vi "HEWH Summary Sheet.vi"(6 "FHD Input":T2={"Calculated Values"={"Draw Cluster - Actual (Gal)"=[], "Mass of water All (lbm)"=[], "Density of hot water All (lbm/gal)"=[], "CpHW (BTU/(lbm °F))"=[], "rho 2 (lb/gal)"=0.0, "rho standby (lb/gal)"=0.0, "rho 24 (lb/gal)"=0.0, "Cp1 (BTU/(lb*F))"=0.0, "Cp2 (BTU/(lb*F))"=0.0, "Cp standby (BTU/(lb*F))"=0.0, "Cp 24 (BTU/(lb*F))"=0.0, "nu_r"=0.0, "Qstby (BTU)"=0.0, "Qhr (BTU/hr)"=0.0, "UA (BTU/(hr*F))"=0.0, "Q (BTU)"=0.0, "Qd (BTU)"=0.0, "Qda (BTU)"=0.0, "QHW67 (BTU)"=0.0, "UEF"=0.0, "Tdel1-Mean Outlet 1st Cluster(°F)"=0.0, "Tin1 - Mean Inlet 1st Cluster (°F)"=0.0, "Cp theoretical (BTU/(lbm °F))"=0.0, "M cluster mass removed (lb)"=0.0, "V1- Vol (Gal)"=0.0, "Test Data -Start to End (Full Index)"=[], "rho_nu (lb/gal)"=0.0, "Density of cold water All (lbm/gal)"=[], "CpUEF (BTU/(lb*F))"=0.0, "QHW (BTU)"=0.0, "QHWD (BTU)"=0.0, "Qdm (BTU)"=0.0, "FHD-After 1 Hour (String)"=[], "Vn"=0.0, "T*avg_del(n)"=0.0, "Max Location"=0, "T*min(n-1)"=0.0, "T*avg_del(n-1)"=0.0, "Temp Greater than T*min(n-1)"=FALSE, "Adjustment Factor"=0.0, "Draw Bonus Volume (gal)"=0.0, "Flow Type - End Condition"=enum."ForcedDrawAfterHour"}, "Sampled Data"={"Cold Water Draw Amounts-(Gal)"=[], "T del_all - Outlet Temps (°F)"=[], "T in_all - Inlet Temps (°F)"=[], "Qsu0 (BTU)"=14385.3, "Qsuf (BTU)"=15959.6, "Tau stby_1 (hr)"=8.4, "T suf(°F)"=125.0, "T su0(°F)"=126.1, "T tstby(°F)"=124.2, "T astby(°F)"=68.8, "T 24(°F)"=123.2, "Qr (BTU)"=7657.9, "T0 (°F)"=124.7, "Tmax1 (°F)"=124.8, "Qe (BTU)"=32770.2, "Qf (BTU)"=0.0, "Tastby2 (°F)"=68.9, "RTD Out Full Data\nSet (Each Draw)"=[], "RTD IN Full Data\nSet (Each Draw)"=[], "Tau stby2 (hr)"=23.406, "Hot Water Draw Amounts-(Gal)"=[], "Cold Flow Rate (GPM)"=[], "Hot Flow Rate (GPM)"=[], "Softw Elapsed Time\n Full Data Set (Each Draw)"=[], "Cold Gal Total Full\nData Set (Each Draw)"=[], "Total Hot Draw Amount (Gal) "=0.0, "Total Cold Draw Amount (Gal)"=0.0, "Qe (Wh)"=0.0, "Hot Gal Total Full\nData Set (Each Draw)"=[]}, "Static Data"={"T-Wh Setpoint (°F)"=125.0, "T-Inlet Setpoint (°F)"=58.0, "T-Ambinet Nominal (°F)"=67.5, "V - Volume of Wh (True)"=46.0}, "Data Indexes"={"Test Start-Full Index (Found)"=0, "Header Length"=0, "Draw Index (Found)"=[], "Nr"=0, "Start Watt Hours"=0.0, "Tsu0 Index (Found)"=0, "Tsf Index (Found)"=0, "Start Energy (BTU-Gas)"=0.0, "Draws in Cluster"=0, "T0 Index-Full Index (Found)"=0, "Non-Draw Index (Found)"=[], "Tmax1 Index (Found)"=0, "Test End-Full Index (Found)"=0, "Heating Index (Found)"=[], "Heating Timestamp"=[], "Non-Draw Timestamp"=[], "Draw Index Timestamp"=[], "Tmax1 Timestamp"=0.0, "Tsu0 Timestamp"=0.0, "Tsf Timestamp"=0.0, "T0 Timestamp"=0.0, "Test End Timestamp"=0.0, "Test Start Timestamp"=0.0, "15 sec after Draw Timestamp"=[], "15 sec after Draw Index"=[], "Tmax1 Occurred During a Draw"=FALSE, "FHD Total Time (Sec)"=0.0, "Draw Pattern"=enum."Very Small Usage", "Standby Valid"=FALSE}, "Raw Data"={"Elapsed Time Index (DBL)"=0, "Software Elapsed Time Index (DBL)"=0, "TC Tree Avg Index (DBL)"=0, "Watt Hours -Wh Index (DBL)"=0, "Energy BTU Index (DBL)"=0, "Totalized Flow Index (DBL)"=0, "Flow Rate Index (DBL)"=0, "Program Status Index (Str)"=0, "RTDin Index (DBL)"=0, "RTDout Index (DBL)"=0, "RTDamb Index (DBL)"=0, "Test Data-Start to End DBL"=[], "Data Type"=enum."GEA Inlet Side Meter", "Heat Source Index (DBL)"=0, "Hot Water Rate GPM (DBL)"=0, "Hot Water Total - GAL (DBL)"=0, "FHD-After 1 hour"=[], "Humidity -% RH (DBL)"=0, "Voltage - V (DBL)"=0, "Draw Count (DBL)"=0, "Elapsed Time Index (Str)"=0, "Software Elapsed Time Index (Str)"=0, "Frequency-Hz (Str)"=0, "RTDin Index (Str)"=0, "RTDout Index (Str)"=0, "RTDamb Index (Str)"=0, "UE (Str)"=0, "LE (Str)"=0, "Compressor (Str)"=0, "Flow Rate Index (Str)"=0, "Hot Water Total - GAL (Str)"=0}, "Tolerance Check (T)=Pass"={"Flow Rate"=FALSE, "Totalized Flow"=FALSE, "Ambient Temp (Full Range)"=FALSE, "Ambient Humidity (Full Range)"=FALSE, "Inlet Temp"=FALSE, "Outlet Temp"=FALSE, "Valid Test"=FALSE, "Individual Totalized Flow"=FALSE, "Data Sheet Check"="", "Inlet Temperature"=[], "Tinlet Max"=[], "Tinlet Min"=[], "Flow Rate Max (Tol)"=[], "Flow Rate Min (Tol)"=[], "Amb Temp Max"=0.0, "Amb Temp Min"=0.0, "Toutlet Max - Draw 1"=0.0, "Humidity Upper Tolerance (%)"=0.0, "Total Volume Tolerance (Gal)"=0.0, "Humidity Lower Tolerance (%)"=0.0, "Flow Rate Max\nPer Draw"=[], "Flow Rate Min\nPer Draw"=[], "Ambient Humidity (Runtime)"=FALSE, "Humidity Avg (Runtime)"=0.0, "Ambient Temp (On-Time AVG)"=FALSE, "Ambient Temp (Off-Time AVG)"=FALSE, "Amb Temp OFF Avg"=0.0, "Amb Temp ON Avg"=0.0, "Voltage (Heating)"=FALSE, "Voltage (Min)"=0.0, "Voltage (Max)"=0.0, "Toutlet Max"=[], "Toutlet Min"=[]}, "Test Information"={"TR Number"="", "Lab ID"="", "Notes/Config"="", "Model Number"="", "Serial Number"="", "Lab Technician"="", "Engineer"="", "Type of Fuel"="", "Samp Received Date"="", "Samp Test Date"="", "Report Date"="", "Rate Input (kW or BTU/hr)"="", "Measured Input (kW or BTU/hr)"="", "Filename"="", "Calibration Information"=[], "Calculator Version"="", "Minimum UEF Per CFR"=0.0, "UEF Report Information"=[], "FHR Report Information"=[], "FHR Front Panel Display"=[], "UEF Front Panel Display"=[], "Draw Outlet Temp Viewer"=[]}} {"Data Indexes"."15 sec after Draw Index" format="%#.2f"; "Data Indexes"."15 sec after Draw Timestamp" format="%#.2f"; "Data Indexes"."Test Start Timestamp" format="%.2f"; "Data Indexes"."Test End Timestamp" format="%.2f"; "Data Indexes"."T0 Timestamp" format="%.2f"; "Data Indexes"."Tsf Timestamp" format="%.2f"; "Data Indexes"."Tsu0 Timestamp" format="%.2f"; "Data Indexes"."Tmax1 Timestamp" format="%.2f"; "Data Indexes"."Draw Index Timestamp" format="%#.2f"; "Data Indexes"."Non-Draw Timestamp" format="%#.2f"; "Data Indexes"."Heating Timestamp" format="%#.2f"; "Data Indexes"."Start Energy (BTU-Gas)" format="%.6f"; "Data Indexes"."Start Watt Hours" format="%.6f"; "Static Data"."V - Volume of Wh (True)" format="%.5f"; "Static Data"."T-Ambinet Nominal (°F)" format="%.5f"; "Static Data"."T-Inlet Setpoint (°F)" format="%.5f"; "Static Data"."T-Wh Setpoint (°F)" format="%.5f"; "Sampled Data"."Qe (Wh)" format="%.5f"; "Sampled Data"."Tau stby2 (hr)" format="%.5f"; "Sampled Data"."Tastby2 (°F)" format="%.5f"; "Sampled Data"."Qf (BTU)" format="%.5f"; "Sampled Data"."Qe (BTU)" format="%.5f"; "Sampled Data"."Tmax1 (°F)" format="%.5f"; "Sampled Data"."T0 (°F)" format="%.5f"; "Sampled Data"."Qr (BTU)" format="%.5f"; "Sampled Data"."T 24(°F)" format="%.5f"; "Sampled Data"."T astby(°F)" format="%.5f"; "Sampled Data"."T tstby(°F)" format="%.5f"; "Sampled Data"."T su0(°F)" format="%.5f"; "Sampled Data"."T suf(°F)" format="%.5f"; "Sampled Data"."Tau stby_1 (hr)" format="%.5f"; "Sampled Data"."Qsuf (BTU)" format="%.5f"; "Sampled Data"."Qsu0 (BTU)" format="%.5f"; "Calculated Values"."Draw Bonus Volume (gal)" format="%.6f"; "Calculated Values"."Adjustment Factor" format="%.6f"; "Calculated Values"."T*avg_del(n-1)" format="%.6f"; "Calculated Values"."T*min(n-1)" format="%.6f"; "Calculated Values"."T*avg_del(n)" format="%.6f"; "Calculated Values"."Vn" format="%.6f"; "Calculated Values"."Qdm (BTU)" format="%.6f"; "Calculated Values"."QHWD (BTU)" format="%.6f"; "Calculated Values"."QHW (BTU)" format="%.6f"; "Calculated Values"."UEF" format="%.6f"; "Calculated Values"."QHW67 (BTU)" format="%.6f"; "Calculated Values"."Qda (BTU)" format="%.6f"; "Calculated Values"."Qd (BTU)" format="%.6f"; "Calculated Values"."Q (BTU)" format="%.6f"; "Calculated Values"."UA (BTU/(hr*F))" format="%.6f"; "Calculated Values"."Qhr (BTU/hr)" format="%.6f"; "Calculated Values"."Qstby (BTU)" format="%.6f"; "Calculated Values"."nu_r" format="%.6f"; "Calculated Values"."CpUEF (BTU/(lb*F))" format="%.6f"; "Calculated Values"."rho_nu (lb/gal)" format="%.6f"; "Calculated Values"."V1- Vol (Gal)" format="%.6f"; "Calculated Values"."M cluster mass removed (lb)" format="%.6f"; "Calculated Values"."Cp theoretical (BTU/(lbm °F))" format="%.6f"; "Calculated Values"."Tin1 - Mean Inlet 1st Cluster (°F)" format="%.6f"; "Calculated Values"."Tdel1-Mean Outlet 1st Cluster(°F)" format="%.6f"; "Calculated Values"."Cp 24 (BTU/(lb*F))" format="%.6f"; "Calculated Values"."Cp standby (BTU/(lb*F))" format="%.6f"; "Calculated Values"."Cp2 (BTU/(lb*F))" format="%.6f"; "Calculated Values"."Cp1 (BTU/(lb*F))" format="%.6f"; "Calculated Values"."rho 24 (lb/gal)" format="%.6f"; "Calculated Values"."rho standby (lb/gal)" format="%.6f"; "Calculated Values"."rho 2 (lb/gal)" format="%.6f"; "Calculated Values"."Density of cold water All (lbm/gal)" format="%#.3g"; "Calculated Values"."CpHW (BTU/(lbm °F))" format="%#.3g"; "Calculated Values"."Density of hot water All (lbm/gal)" format="%#.3g"; "Calculated Values"."Mass of water All (lbm)" format="%#.3f"}, 8 "error in (no error)":errorcluster, 10 "UEF Calculated Values Input":T2={"Calculated Values"={"Draw Cluster - Actual (Gal)"=[], "Mass of water All (lbm)"=[], "Density of hot water All (lbm/gal)"=[], "CpHW (BTU/(lbm °F))"=[], "rho 2 (lb/gal)"=0.0, "rho standby (lb/gal)"=0.0, "rho 24 (lb/gal)"=0.0, "Cp1 (BTU/(lb*F))"=0.0, "Cp2 (BTU/(lb*F))"=0.0, "Cp standby (BTU/(lb*F))"=0.0, "Cp 24 (BTU/(lb*F))"=0.0, "nu_r"=0.0, "Qstby (BTU)"=0.0, "Qhr (BTU/hr)"=0.0, "UA (BTU/(hr*F))"=0.0, "Q (BTU)"=0.0, "Qd (BTU)"=0.0, "Qda (BTU)"=0.0, "QHW67 (BTU)"=0.0, "UEF"=0.0, "Tdel1-Mean Outlet 1st Cluster(°F)"=0.0, "Tin1 - Mean Inlet 1st Cluster (°F)"=0.0, "Cp theoretical (BTU/(lbm °F))"=0.0, "M cluster mass removed (lb)"=0.0, "V1- Vol (Gal)"=0.0, "Test Data -Start to End (Full Index)"=[], "rho_nu (lb/gal)"=0.0, "Density of cold water All (lbm/gal)"=[], "CpUEF (BTU/(lb*F))"=0.0, "QHW (BTU)"=0.0, "QHWD (BTU)"=0.0, "Qdm (BTU)"=0.0, "FHD-After 1 Hour (String)"=[], "Vn"=0.0, "T*avg_del(n)"=0.0, "Max Location"=0, "T*min(n-1)"=0.0, "T*avg_del(n-1)"=0.0, "Temp Greater than T*min(n-1)"=FALSE, "Adjustment Factor"=0.0, "Draw Bonus Volume (gal)"=0.0, "Flow Type - End Condition"=enum."ForcedDrawAfterHour"}, "Sampled Data"={"Cold Water Draw Amounts-(Gal)"=[], "T del_all - Outlet Temps (°F)"=[], "T in_all - Inlet Temps (°F)"=[], "Qsu0 (BTU)"=14385.3, "Qsuf (BTU)"=15959.6, "Tau stby_1 (hr)"=8.4, "T suf(°F)"=125.0, "T su0(°F)"=126.1, "T tstby(°F)"=124.2, "T astby(°F)"=68.8, "T 24(°F)"=123.2, "Qr (BTU)"=7657.9, "T0 (°F)"=124.7, "Tmax1 (°F)"=124.8, "Qe (BTU)"=32770.2, "Qf (BTU)"=0.0, "Tastby2 (°F)"=68.9, "RTD Out Full Data\nSet (Each Draw)"=[], "RTD IN Full Data\nSet (Each Draw)"=[], "Tau stby2 (hr)"=23.406, "Hot Water Draw Amounts-(Gal)"=[], "Cold Flow Rate (GPM)"=[], "Hot Flow Rate (GPM)"=[], "Softw Elapsed Time\n Full Data Set (Each Draw)"=[], "Cold Gal Total Full\nData Set (Each Draw)"=[], "Total Hot Draw Amount (Gal) "=0.0, "Total Cold Draw Amount (Gal)"=0.0, "Qe (Wh)"=0.0, "Hot Gal Total Full\nData Set (Each Draw)"=[]}, "Static Data"={"T-Wh Setpoint (°F)"=125.0, "T-Inlet Setpoint (°F)"=58.0, "T-Ambinet Nominal (°F)"=67.5, "V - Volume of Wh (True)"=46.0}, "Data Indexes"={"Test Start-Full Index (Found)"=0, "Header Length"=0, "Draw Index (Found)"=[], "Nr"=0, "Start Watt Hours"=0.0, "Tsu0 Index (Found)"=0, "Tsf Index (Found)"=0, "Start Energy (BTU-Gas)"=0.0, "Draws in Cluster"=0, "T0 Index-Full Index (Found)"=0, "Non-Draw Index (Found)"=[], "Tmax1 Index (Found)"=0, "Test End-Full Index (Found)"=0, "Heating Index (Found)"=[], "Heating Timestamp"=[], "Non-Draw Timestamp"=[], "Draw Index Timestamp"=[], "Tmax1 Timestamp"=0.0, "Tsu0 Timestamp"=0.0, "Tsf Timestamp"=0.0, "T0 Timestamp"=0.0, "Test End Timestamp"=0.0, "Test Start Timestamp"=0.0, "15 sec after Draw Timestamp"=[], "15 sec after Draw Index"=[], "Tmax1 Occurred During a Draw"=FALSE, "FHD Total Time (Sec)"=0.0, "Draw Pattern"=enum."Very Small Usage", "Standby Valid"=FALSE}, "Raw Data"={"Elapsed Time Index (DBL)"=0, "Software Elapsed Time Index (DBL)"=0, "TC Tree Avg Index (DBL)"=0, "Watt Hours -Wh Index (DBL)"=0, "Energy BTU Index (DBL)"=0, "Totalized Flow Index (DBL)"=0, "Flow Rate Index (DBL)"=0, "Program Status Index (Str)"=0, "RTDin Index (DBL)"=0, "RTDout Index (DBL)"=0, "RTDamb Index (DBL)"=0, "Test Data-Start to End DBL"=[], "Data Type"=enum."GEA Inlet Side Meter", "Heat Source Index (DBL)"=0, "Hot Water Rate GPM (DBL)"=0, "Hot Water Total - GAL (DBL)"=0, "FHD-After 1 hour"=[], "Humidity -% RH (DBL)"=0, "Voltage - V (DBL)"=0, "Draw Count (DBL)"=0, "Elapsed Time Index (Str)"=0, "Software Elapsed Time Index (Str)"=0, "Frequency-Hz (Str)"=0, "RTDin Index (Str)"=0, "RTDout Index (Str)"=0, "RTDamb Index (Str)"=0, "UE (Str)"=0, "LE (Str)"=0, "Compressor (Str)"=0, "Flow Rate Index (Str)"=0, "Hot Water Total - GAL (Str)"=0}, "Tolerance Check (T)=Pass"={"Flow Rate"=FALSE, "Totalized Flow"=FALSE, "Ambient Temp (Full Range)"=FALSE, "Ambient Humidity (Full Range)"=FALSE, "Inlet Temp"=FALSE, "Outlet Temp"=FALSE, "Valid Test"=FALSE, "Individual Totalized Flow"=FALSE, "Data Sheet Check"="", "Inlet Temperature"=[], "Tinlet Max"=[], "Tinlet Min"=[], "Flow Rate Max (Tol)"=[], "Flow Rate Min (Tol)"=[], "Amb Temp Max"=0.0, "Amb Temp Min"=0.0, "Toutlet Max - Draw 1"=0.0, "Humidity Upper Tolerance (%)"=0.0, "Total Volume Tolerance (Gal)"=0.0, "Humidity Lower Tolerance (%)"=0.0, "Flow Rate Max\nPer Draw"=[], "Flow Rate Min\nPer Draw"=[], "Ambient Humidity (Runtime)"=FALSE, "Humidity Avg (Runtime)"=0.0, "Ambient Temp (On-Time AVG)"=FALSE, "Ambient Temp (Off-Time AVG)"=FALSE, "Amb Temp OFF Avg"=0.0, "Amb Temp ON Avg"=0.0, "Voltage (Heating)"=FALSE, "Voltage (Min)"=0.0, "Voltage (Max)"=0.0, "Toutlet Max"=[], "Toutlet Min"=[]}, "Test Information"={"TR Number"="", "Lab ID"="", "Notes/Config"="", "Model Number"="", "Serial Number"="", "Lab Technician"="", "Engineer"="", "Type of Fuel"="", "Samp Received Date"="", "Samp Test Date"="", "Report Date"="", "Rate Input (kW or BTU/hr)"="", "Measured Input (kW or BTU/hr)"="", "Filename"="", "Calibration Information"=[], "Calculator Version"="", "Minimum UEF Per CFR"=0.0, "UEF Report Information"=[], "FHR Report Information"=[], "FHR Front Panel Display"=[], "UEF Front Panel Display"=[], "Draw Outlet Temp Viewer"=[]}} {"Data Indexes"."15 sec after Draw Index" format="%#.2f"; "Data Indexes"."15 sec after Draw Timestamp" format="%#.2f"; "Data Indexes"."Test Start Timestamp" format="%.2f"; "Data Indexes"."Test End Timestamp" format="%.2f"; "Data Indexes"."T0 Timestamp" format="%.2f"; "Data Indexes"."Tsf Timestamp" format="%.2f"; "Data Indexes"."Tsu0 Timestamp" format="%.2f"; "Data Indexes"."Tmax1 Timestamp" format="%.2f"; "Data Indexes"."Draw Index Timestamp" format="%#.2f"; "Data Indexes"."Non-Draw Timestamp" format="%#.2f"; "Data Indexes"."Heating Timestamp" format="%#.2f"; "Data Indexes"."Start Energy (BTU-Gas)" format="%.6f"; "Data Indexes"."Start Watt Hours" format="%.6f"; "Static Data"."V - Volume of Wh (True)" format="%.5f"; "Static Data"."T-Ambinet Nominal (°F)" format="%.5f"; "Static Data"."T-Inlet Setpoint (°F)" format="%.5f"; "Static Data"."T-Wh Setpoint (°F)" format="%.5f"; "Sampled Data"."Qe (Wh)" format="%.5f"; "Sampled Data"."Tau stby2 (hr)" format="%.5f"; "Sampled Data"."Tastby2 (°F)" format="%.5f"; "Sampled Data"."Qf (BTU)" format="%.5f"; "Sampled Data"."Qe (BTU)" format="%.5f"; "Sampled Data"."Tmax1 (°F)" format="%.5f"; "Sampled Data"."T0 (°F)" format="%.5f"; "Sampled Data"."Qr (BTU)" format="%.5f"; "Sampled Data"."T 24(°F)" format="%.5f"; "Sampled Data"."T astby(°F)" format="%.5f"; "Sampled Data"."T tstby(°F)" format="%.5f"; "Sampled Data"."T su0(°F)" format="%.5f"; "Sampled Data"."T suf(°F)" format="%.5f"; "Sampled Data"."Tau stby_1 (hr)" format="%.5f"; "Sampled Data"."Qsuf (BTU)" format="%.5f"; "Sampled Data"."Qsu0 (BTU)" format="%.5f"; "Calculated Values"."Draw Bonus Volume (gal)" format="%.6f"; "Calculated Values"."Adjustment Factor" format="%.6f"; "Calculated Values"."T*avg_del(n-1)" format="%.6f"; "Calculated Values"."T*min(n-1)" format="%.6f"; "Calculated Values"."T*avg_del(n)" format="%.6f"; "Calculated Values"."Vn" format="%.6f"; "Calculated Values"."Qdm (BTU)" format="%.6f"; "Calculated Values"."QHWD (BTU)" format="%.6f"; "Calculated Values"."QHW (BTU)" format="%.6f"; "Calculated Values"."UEF" format="%.6f"; "Calculated Values"."QHW67 (BTU)" format="%.6f"; "Calculated Values"."Qda (BTU)" format="%.6f"; "Calculated Values"."Qd (BTU)" format="%.6f"; "Calculated Values"."Q (BTU)" format="%.6f"; "Calculated Values"."UA (BTU/(hr*F))" format="%.6f"; "Calculated Values"."Qhr (BTU/hr)" format="%.6f"; "Calculated Values"."Qstby (BTU)" format="%.6f"; "Calculated Values"."nu_r" format="%.6f"; "Calculated Values"."CpUEF (BTU/(lb*F))" format="%.6f"; "Calculated Values"."rho_nu (lb/gal)" format="%.6f"; "Calculated Values"."V1- Vol (Gal)" format="%.6f"; "Calculated Values"."M cluster mass removed (lb)" format="%.6f"; "Calculated Values"."Cp theoretical (BTU/(lbm °F))" format="%.6f"; "Calculated Values"."Tin1 - Mean Inlet 1st Cluster (°F)" format="%.6f"; "Calculated Values"."Tdel1-Mean Outlet 1st Cluster(°F)" format="%.6f"; "Calculated Values"."Cp 24 (BTU/(lb*F))" format="%.6f"; "Calculated Values"."Cp standby (BTU/(lb*F))" format="%.6f"; "Calculated Values"."Cp2 (BTU/(lb*F))" format="%.6f"; "Calculated Values"."Cp1 (BTU/(lb*F))" format="%.6f"; "Calculated Values"."rho 24 (lb/gal)" format="%.6f"; "Calculated Values"."rho standby (lb/gal)" format="%.6f"; "Calculated Values"."rho 2 (lb/gal)" format="%.6f"; "Calculated Values"."Density of cold water All (lbm/gal)" format="%#.3g"; "Calculated Values"."CpHW (BTU/(lbm °F))" format="%#.3g"; "Calculated Values"."Density of hot water All (lbm/gal)" format="%#.3g"; "Calculated Values"."Mass of water All (lbm)" format="%#.3f"}, 11 "report in":refnum<class "NI_report.lvclass">) -> (0 "error out":errorcluster, 3 "report out":refnum<class "NI_report.lvclass">)   [LabVIEW 2023]
uses:
  <vilib>/Utility/NIReport.llb/NI_report.lvclass
  Type Definitions/UEF Constants.ctl
  Type Definitions/HEWH Draw Stats.ctl
  Type Definitions/HEWH FHR Draw Type.ctl
  Type Definitions/FHR Bins.ctl
  Type Definitions/HEWH Meter Type.ctl
  <vilib>/addons/_office/_exclsub.llb/font.ctl
  <vilib>/Analysis/baseanly.llb/Mean (DBL).vi
  <vilib>/addons/_office/NI_ReportGenerationToolkit.lvlib
  <vilib>/Utility/NIReport.llb/Excel/NI_Excel.lvclass
  <vilib>/Analysis/NI_AALBase.lvlib
panel:
  out "Draw Pattern":T1
  # "FHR"
  # "FHR"
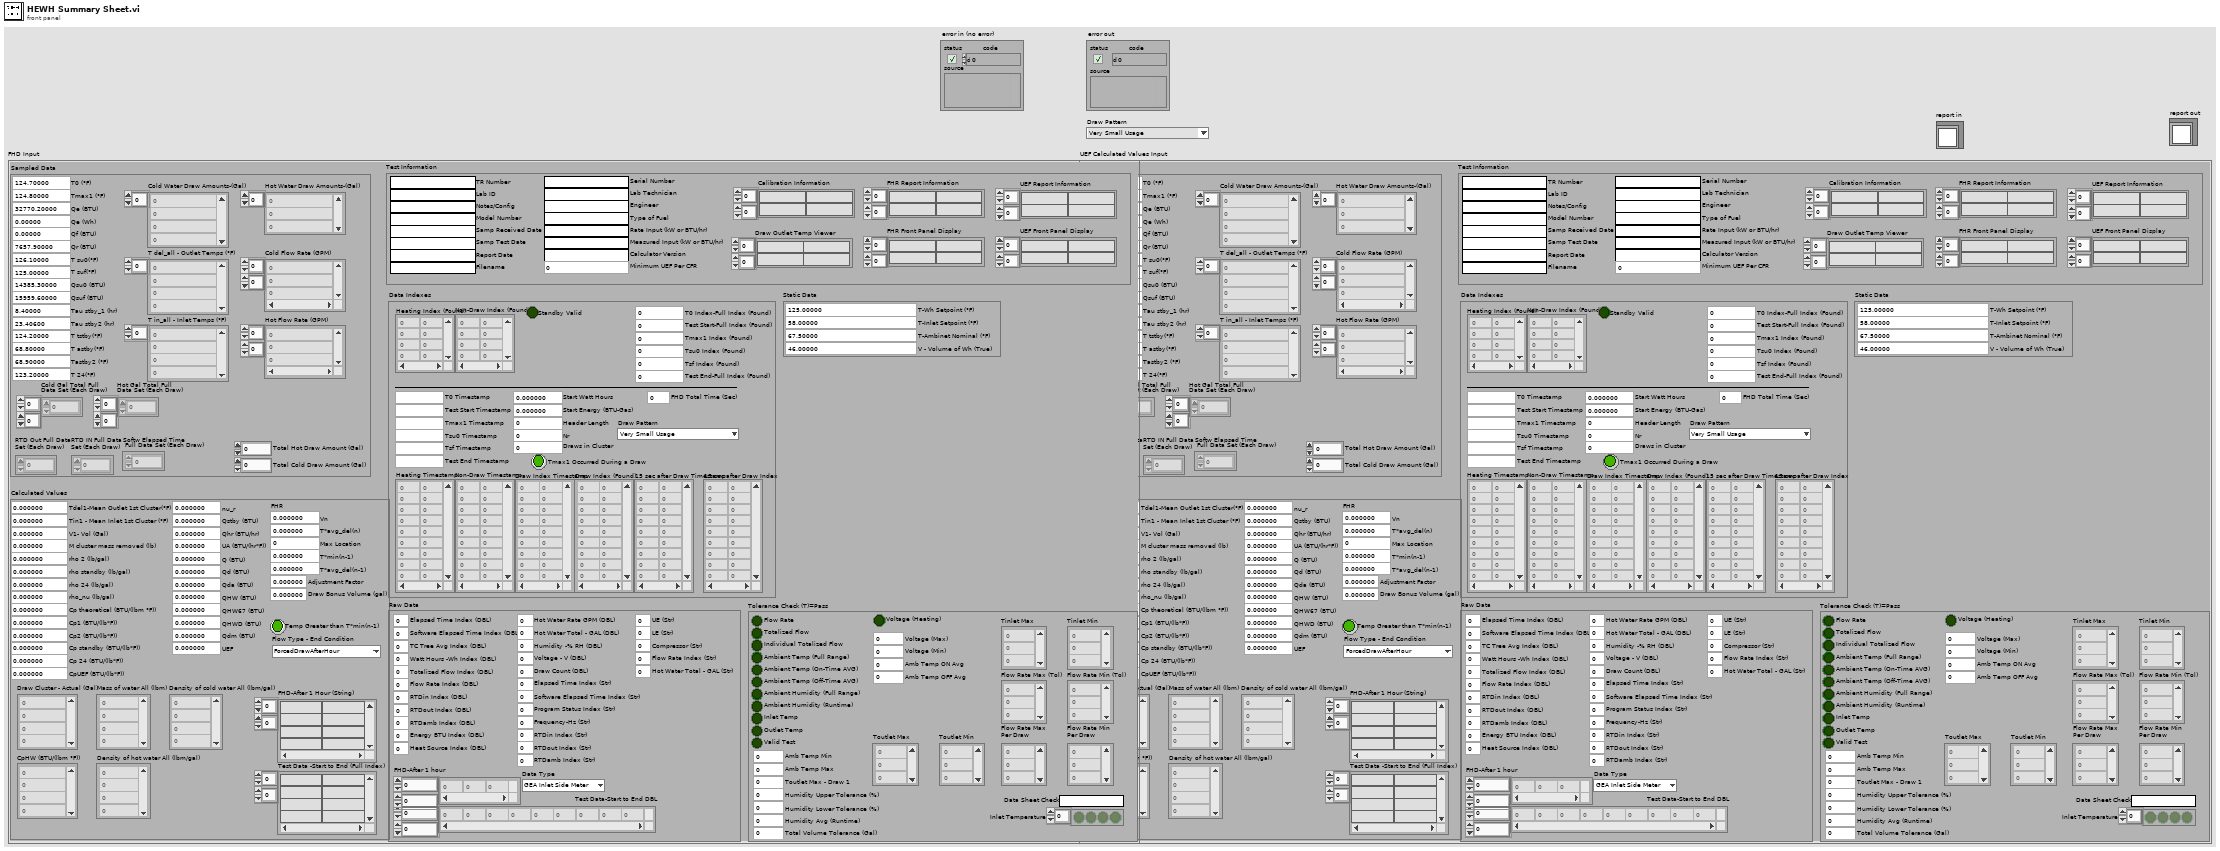
[diagram p1: front panel]
types:
  T1 = typedef "FHR Bins.ctl" = enum16{"Very Small Usage", "Low Usage", "Medium Usage", "High Usage", "Undefined"}
  T2 = typedef "UEF Constants.ctl" = cluster{"Calculated Values":T3, "Sampled Data":cluster{"Cold Water Draw Amounts-(Gal)":dbl[], "T del_all - Outlet Temps (°F)":dbl[], "T in_all - Inlet Temps (°F)":dbl[], "Qsu0 (BTU)":dbl, "Qsuf (BTU)":dbl, "Tau stby_1 (hr)":dbl, "T suf(°F)":dbl, "T su0(°F)":dbl, "T tstby(°F)":dbl, "T astby(°F)":dbl, "T 24(°F)":dbl, "Qr (BTU)":dbl, "T0 (°F)":dbl, "Tmax1 (°F)":dbl, "Qe (BTU)":dbl, "Qf (BTU)":dbl, "Tastby2 (°F)":dbl, "RTD Out Full Data\nSet (Each Draw)":dbl[][], "RTD IN Full Data\nSet (Each Draw)":dbl[][], "Tau stby2 (hr)":dbl, "Hot Water Draw Amounts-(Gal)":dbl[], "Cold Flow Rate (GPM)":dbl[][], "Hot Flow Rate (GPM)":dbl[][], "Softw Elapsed Time\n Full Data Set (Each Draw)":dbl[][], "Cold Gal Total Full\nData Set (Each Draw)":dbl[][], "Total Hot Draw Amount (Gal) ":dbl, "Total Cold Draw Amount (Gal)":dbl, "Qe (Wh)":dbl, "Hot Gal Total Full\nData Set (Each Draw)":dbl[][]}, "Static Data":cluster{"T-Wh Setpoint (°F)":dbl, "T-Inlet Setpoint (°F)":dbl, "T-Ambinet Nominal (°F)":dbl, "V - Volume of Wh (True)":dbl}, "Data Indexes":cluster{"Test Start-Full Index (Found)":i32, "Header Length":i32, "Draw Index (Found)":i32[][], "Nr":i32, "Start Watt Hours":dbl, "Tsu0 Index (Found)":i32, "Tsf Index (Found)":i32, "Start Energy (BTU-Gas)":dbl, "Draws in Cluster":i32, "T0 Index-Full Index (Found)":i32, "Non-Draw Index (Found)":i32[][], "Tmax1 Index (Found)":i32, "Test End-Full Index (Found)":i32, "Heating Index (Found)":i32[][], "Heating Timestamp":dbl[][], "Non-Draw Timestamp":dbl[][], "Draw Index Timestamp":dbl[][], "Tmax1 Timestamp":dbl, "Tsu0 Timestamp":dbl, "Tsf Timestamp":dbl, "T0 Timestamp":dbl, "Test End Timestamp":dbl, "Test Start Timestamp":dbl, "15 sec after Draw Timestamp":dbl[][], "15 sec after Draw Index":dbl[][], "Tmax1 Occurred During a Draw":bool, "FHD Total Time (Sec)":dbl, "Draw Pattern":T1, "Standby Valid":bool}, "Raw Data":cluster{"Elapsed Time Index (DBL)":i32, "Software Elapsed Time Index (DBL)":i32, "TC Tree Avg Index (DBL)":i32, "Watt Hours -Wh Index (DBL)":i32, "Energy BTU Index (DBL)":i32, "Totalized Flow Index (DBL)":i32, "Flow Rate Index (DBL)":i32, "Program Status Index (Str)":i32, "RTDin Index (DBL)":i32, "RTDout Index (DBL)":i32, "RTDamb Index (DBL)":i32, "Test Data-Start to End DBL":dbl[][], "Data Type":T5, "Heat Source Index (DBL)":i32, "Hot Water Rate GPM (DBL)":i32, "Hot Water Total - GAL (DBL)":i32, "FHD-After 1 hour":dbl[][], "Humidity -% RH (DBL)":i32, "Voltage - V (DBL)":i32, "Draw Count (DBL)":i32, "Elapsed Time Index (Str)":i32, "Software Elapsed Time Index (Str)":i32, "Frequency-Hz (Str)":i32, "RTDin Index (Str)":i32, "RTDout Index (Str)":i32, "RTDamb Index (Str)":i32, "UE (Str)":i32, "LE (Str)":i32, "Compressor (Str)":i32, "Flow Rate Index (Str)":i32, "Hot Water Total - GAL (Str)":i32}, "Tolerance Check (T)=Pass":cluster{"Flow Rate":bool, "Totalized Flow":bool, "Ambient Temp (Full Range)":bool, "Ambient Humidity (Full Range)":bool, "Inlet Temp":bool, "Outlet Temp":bool, "Valid Test":bool, "Individual Totalized Flow":bool, "Data Sheet Check":string, "Inlet Temperature":bool[], "Tinlet Max":dbl[], "Tinlet Min":dbl[], "Flow Rate Max (Tol)":dbl[], "Flow Rate Min (Tol)":dbl[], "Amb Temp Max":dbl, "Amb Temp Min":dbl, "Toutlet Max - Draw 1":dbl, "Humidity Upper Tolerance (%)":dbl, "Total Volume Tolerance (Gal)":dbl, "Humidity Lower Tolerance (%)":dbl, "Flow Rate Max\nPer Draw":dbl[], "Flow Rate Min\nPer Draw":dbl[], "Ambient Humidity (Runtime)":bool, "Humidity Avg (Runtime)":dbl, "Ambient Temp (On-Time AVG)":bool, "Ambient Temp (Off-Time AVG)":bool, "Amb Temp OFF Avg":dbl, "Amb Temp ON Avg":dbl, "Voltage (Heating)":bool, "Voltage (Min)":dbl, "Voltage (Max)":dbl, "Toutlet Max":dbl[], "Toutlet Min":dbl[]}, "Test Information":cluster{"TR Number":string, "Lab ID":string, "Notes/Config":string, "Model Number":string, "Serial Number":string, "Lab Technician":string, "Engineer":string, "Type of Fuel":string, "Samp Received Date":string, "Samp Test Date":string, "Report Date":string, "Rate Input (kW or BTU/hr)":string, "Measured Input (kW or BTU/hr)":string, "Filename":string, "Calibration Information":string[][], "Calculator Version":string, "Minimum UEF Per CFR":dbl, "UEF Report Information":string[][], "FHR Report Information":string[][], "FHR Front Panel Display":string[][], "UEF Front Panel Display":string[][], "Draw Outlet Temp Viewer":string[][]}}
  T3 = typedef "HEWH Draw Stats.ctl" = cluster{"Draw Cluster - Actual (Gal)":dbl[], "Mass of water All (lbm)":dbl[], "Density of hot water All (lbm/gal)":dbl[], "CpHW (BTU/(lbm °F))":dbl[], "rho 2 (lb/gal)":dbl, "rho standby (lb/gal)":dbl, "rho 24 (lb/gal)":dbl, "Cp1 (BTU/(lb*F))":dbl, "Cp2 (BTU/(lb*F))":dbl, "Cp standby (BTU/(lb*F))":dbl, "Cp 24 (BTU/(lb*F))":dbl, "nu_r":dbl, "Qstby (BTU)":dbl, "Qhr (BTU/hr)":dbl, "UA (BTU/(hr*F))":dbl, "Q (BTU)":dbl, "Qd (BTU)":dbl, "Qda (BTU)":dbl, "QHW67 (BTU)":dbl, "UEF":dbl, "Tdel1-Mean Outlet 1st Cluster(°F)":dbl, "Tin1 - Mean Inlet 1st Cluster (°F)":dbl, "Cp theoretical (BTU/(lbm °F))":dbl, "M cluster mass removed (lb)":dbl, "V1- Vol (Gal)":dbl, "Test Data -Start to End (Full Index)":string[][], "rho_nu (lb/gal)":dbl, "Density of cold water All (lbm/gal)":dbl[], "CpUEF (BTU/(lb*F))":dbl, "QHW (BTU)":dbl, "QHWD (BTU)":dbl, "Qdm (BTU)":dbl, "FHD-After 1 Hour (String)":string[][], "Vn":dbl, "T*avg_del(n)":dbl, "Max Location":i32, "T*min(n-1)":dbl, "T*avg_del(n-1)":dbl, "Temp Greater than T*min(n-1)":bool, "Adjustment Factor":dbl, "Draw Bonus Volume (gal)":dbl, "Flow Type - End Condition":T4}
  T4 = typedef "HEWH FHR Draw Type.ctl" = enum16{"ForcedDrawAfterHour", "HeatingCutoffBeforeHour"}
  T5 = typedef "HEWH Meter Type.ctl" = enum16{"GEA Inlet Side Meter", "GEA Outlet Side Meter", "CSA Inlet Side Meter"}
  T6 = typedef "NI_ReportGenerationToolkit.lvlib/font.ctl" = cluster{"font name":string, "font size":dbl, "bold":u16, "italic":u16, "underline":u16, "strike through":u16, "font color":u32}
  T7 = cluster{"on/off":bool, "weight":i32, "color":u32}
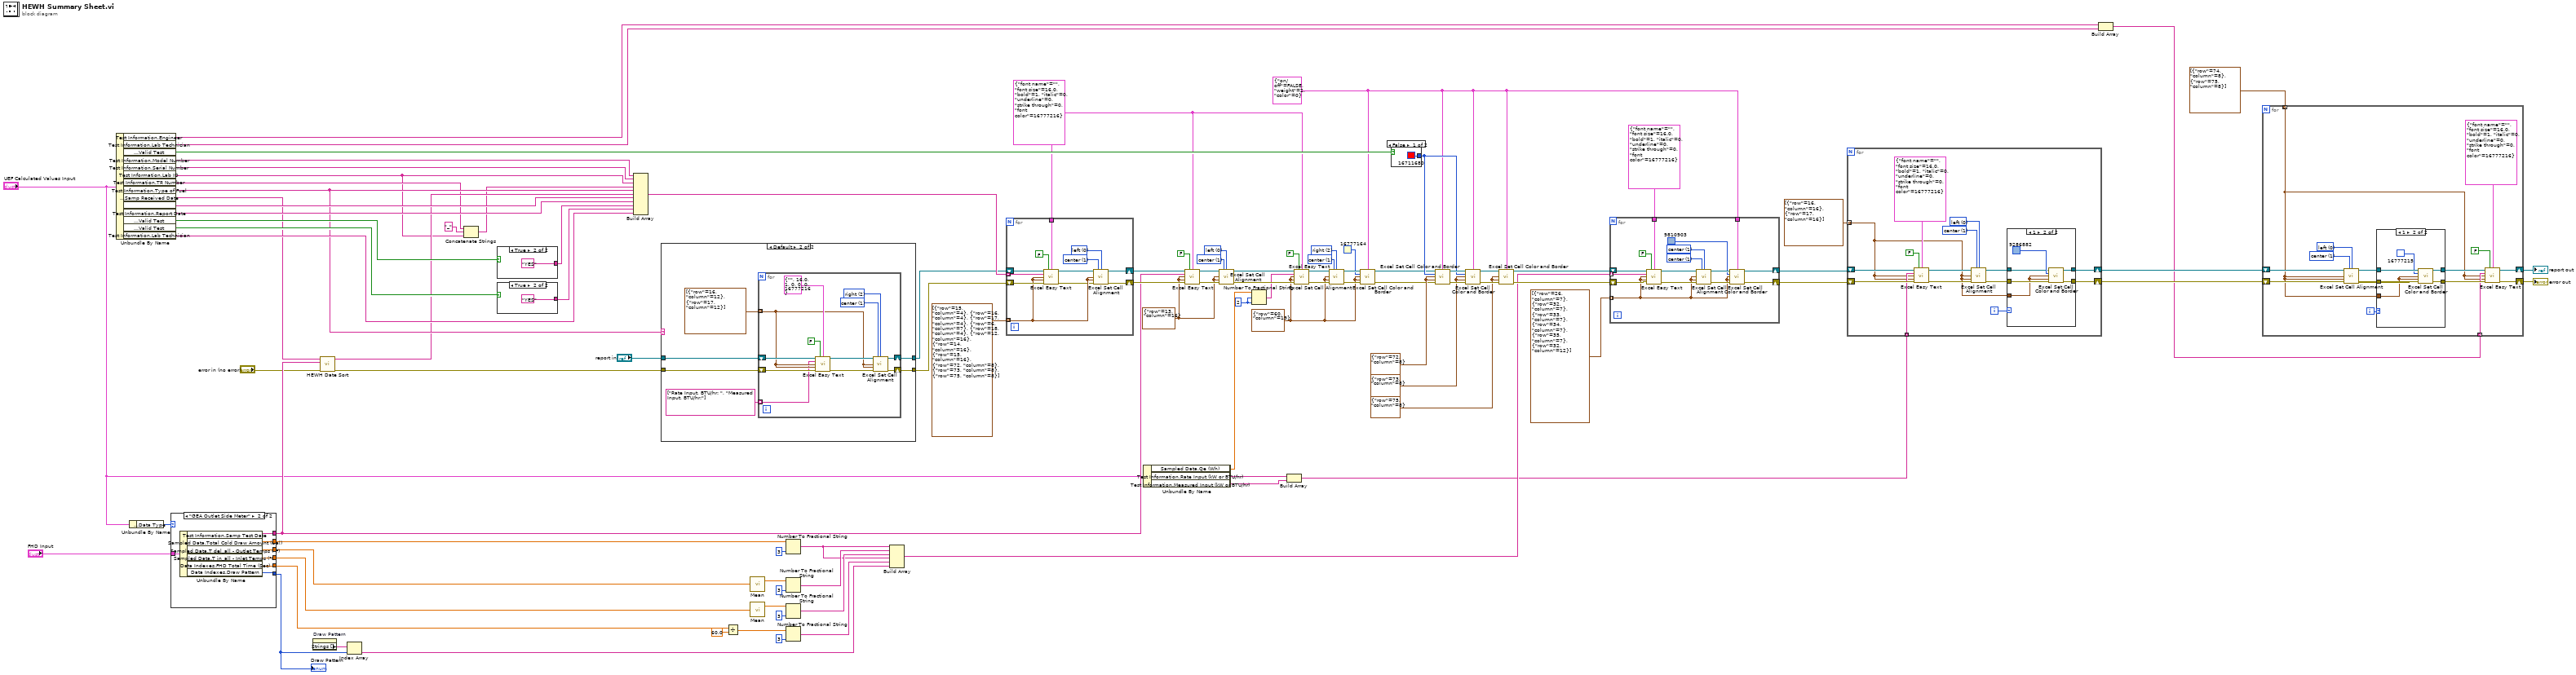
[diagram p0: block diagram]
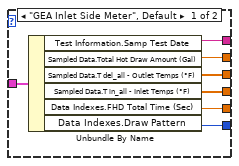
[diagram p2: hidden frame]
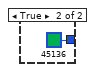
[diagram p6: hidden frame]
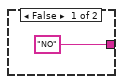
[diagram p7: hidden frame]
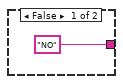
[diagram p8: hidden frame]
diagram:
  w11 = i16 2 ("precision (6)")
  w4 = cluster{"row":i32, "column":i32} {"row"=60, "column"=19} ("start (-1, -1)")
  w20 = 2 items=["left", "center", "right"] ("horizontal alignment (left)")
  w19 = 1 items=["top", "center", "bottom"] ("vertical alignment (top)")
  w33 = cluster{"row":i32, "column":i32} {"row"=13, "column"=16} ("start (-1, -1)")
  w37 = 0 items=["left", "center", "right"] ("horizontal alignment (left)")
  w38 = 1 items=["top", "center", "bottom"] ("vertical alignment (top)")
  w81 = cluster{"row":i32, "column":i32} {"row"=75, "column"=8} ("start (-1, -1)")
  w6 = T7 {"on/off"=FALSE, "weight"=2, "color"=0} ("outside border")
  w85 = cluster{"row":i32, "column":i32} {"row"=73, "column"=8} ("start (-1, -1)")
  w86 = cluster{"row":i32, "column":i32} {"row"=72, "column"=8} ("start (-1, -1)")
  w15 = T6 {"font name"="", "font size"=16.0, "bold"=1, "italic"=0, "underline"=0, "strike through"=0, "font color"=16777216} ("font")
  n1 = Unbundle By Name("UEF Calculated Values Input") -> ("Test Information.Engineer"=w43:string, "Test Information.Lab Technician"=w42:string, "Tolerance Check (T)=Pass.Valid Test"=w87:bool, "Test Information.Model Number"=w100:string, "Test Information.Serial Number"=w99:string, "Test Information.Lab ID"=w23:string, "Test Information.TR Number"=w25:string, "Test Information.Type of Fuel"=w67:string, "Test Information.Samp Received Date"=w32:string, "Test Information.Samp Test Date"=w97:string, "Test Information.Report Date"=w96:string, "Tolerance Check (T)=Pass.Valid Test"=w94:bool, "Tolerance Check (T)=Pass.Valid Test"=w92:bool, "Test Information.Lab Technician"=w84:string)
  n2 = Unbundle By Name("UEF Calculated Values Input") -> ("Raw Data.Data Type"=w26:T5)
  n3 = case shown="\"GEA Outlet Side Meter\"" w26 {
    tunnel: "FHD Input" -> [w107 w114]
    tunnel: [w106 w109] -> w79
    tunnel: [w105 w110] -> w77
    tunnel: [w104 w111] -> w76
    tunnel: [w103 w112] -> w75
    tunnel: [w102 w108] -> w2
    tunnel: [w101 w113] -> w31
    frame "GEA Inlet Side Meter", Default {
      n4 = Unbundle By Name(w107) -> ("Test Information.Samp Test Date"=w101:string, "Sampled Data.Total Hot Draw Amount (Gal)"=w103:dbl, "Sampled Data.T del_all - Outlet Temps (°F)"=w104:dbl[], "Sampled Data.T in_all - Inlet Temps (°F)"=w105:dbl[], "Data Indexes.FHD Total Time (Sec)"=w106:dbl, "Data Indexes.Draw Pattern"=w102:T1)
    }
    frame "GEA Outlet Side Meter" {
      n5 = Unbundle By Name(w114) -> ("Test Information.Samp Test Date"=w113:string, "Sampled Data.Total Cold Draw Amount (Gal)"=w112:dbl, "Sampled Data.T del_all - Outlet Temps (°F)"=w111:dbl[], "Sampled Data.T in_all - Inlet Temps (°F)"=w110:dbl[], "Data Indexes.FHD Total Time (Sec)"=w109:dbl, "Data Indexes.Draw Pattern"=w108:T1)
    }
  }
  "Draw Pattern" <- w2
  n6 = property on="Draw Pattern" class="Enum (strict)"() -> ("Strings []"=w3:string[])  [unwired: 2 in, 2 out]
  n7 = call "HEWH Date Sort.vi"("error in (no error)"="error in (no error)", "FHR Test Date"=w31, "24 Hour Test Date"=w32) -> ("error out"=w28:errorcluster, "Earliest Date"=w30:string)  [unwired: 7 in]
  n8 = Index Array(array=w3, index=w2) -> (element=w1:string)
  n9 = Concatenate Strings(w25, "_" ("string"), w23) -> (w22:string)
  n10 = case shown="True" w94 {
    tunnel: ["NO" "YES"] -> w93
    frame False {
    }
    frame True {
    }
  }
  n11 = case shown="True" w92 {
    tunnel: ["NO" "YES"] -> w91
    frame False {
    }
    frame True {
    }
  }
  n12 = Build Array(w100, w99, w23, w22, w67, w30, w97, w96, w93, w91, w84) -> (w98:string[])
  n13 = case shown="Default" w67 {
    tunnel: "report in" -> [w119 w126]
    tunnel: w28 -> [w120 w125]
    tunnel: [w119 w124] -> w57
    tunnel: [w120 w123] -> w56
    frame "Electric" {
    }
    frame Default {
      n14 = for {
        tunnel: cluster{"row":i32, "column":i32}[] [{"row"=16, "column"=12}, {"row"=17, "column"=12}] -> [w128] mode=indexing
        shift-right: [w131] -> w124
        shift-left: w126 -> [w133]
        shift-right: [w130] -> w123
        shift-left: w125 -> [w132]
        tunnel: string[] ["Rate Input, BTU/hr: ", "Measured Input, BTU/hr:"] -> [w127] mode=indexing
        w135 = 2 items=["left", "center", "right"] ("horizontal alignment (left)")
        w136 = 1 items=["top", "center", "bottom"] ("vertical alignment (top)")
        n15 = call <vilib>:"Excel Easy Text.vi"("report in"=w133, "border? (F)"=FALSE, "font"=T6 {"font name"="", "font size"=16.0, "bold"=1, "italic"=0, "underline"=0, "strike through"=0, "font color"=16777216}, "text"=w127, "start (-1, -1)"=w128, "end (-1, -1)"=w128, "error in (no error)"=w132) -> ("report out"=w137:refnum<class "NI_report.lvclass">, "error out"=w138:errorcluster)  [unwired: 4 in, 3 out]
        n16 = call <vilib>:"Excel Set Cell Alignment.vi"("report in"=w137, "vertical alignment (top)"=w136, "horizontal alignment (left)"=w135, "start (-1, -1)"=w128, "end (-1, -1)"=w128, "error in (no error)"=w138) -> ("report out"=w131:refnum<class "NI_report.lvclass">, "error out"=w130:errorcluster)  [unwired: 8 in]
      }
    }
  }
  n17 = Divide(x=w79, y=60.0) -> (x/y=w68:dbl)
  n18 = call-poly <vilib>:"Mean.vi"("X"=w76) -> ("mean"=w72:dbl)  [unwired: 1 out]
  n19 = call-poly <vilib>:"Mean.vi"("X"=w77) -> ("mean"=w70:dbl)  [unwired: 1 out]
  n20 = Number To Fractional String(number=w75, precision (6)=i16 3) -> (F-format string=w49:string)  [unwired: 2 in]
  n21 = Number To Fractional String(number=w72, precision (6)=i16 3) -> (F-format string=w62:string)  [unwired: 2 in]
  n22 = Number To Fractional String(number=w70, precision (6)=i16 3) -> (F-format string=w61:string)  [unwired: 2 in]
  n23 = Number To Fractional String(number=w68, precision (6)=i16 3) -> (F-format string=w60:string)  [unwired: 2 in]
  n24 = Build Array(w49, w62, w61, w49, w60, w1) -> (w59:string[])
  n25 = for {
    tunnel: w15 -> [w147]
    tunnel: w98 -> [w142] mode=indexing
    shift-right: [w146] -> w35
    shift-left: w56 -> [w145]
    shift-right: [w143] -> w34
    shift-left: w57 -> [w144]
    tunnel: cluster{"row":i32, "column":i32}[] [{"row"=15, "column"=4}, {"row"=16, "column"=4}, {"row"=17, "column"=4}, {"row"=6, "column"=7}, {"row"=18, "column"=4}, {"row"=12, "column"=16}, {"row"=14, "column"=16}, {"row"=15, "column"=16}, {"row"=72, "column"=8}, {"row"=73, "column"=8}, {"row"=75, "column"=8}] -> [w141] mode=indexing
    w149 = 0 items=["left", "center", "right"] ("horizontal alignment (left)")
    w148 = 1 items=["top", "center", "bottom"] ("vertical alignment (top)")
    n26 = call <vilib>:"Excel Easy Text.vi"("report in"=w144, "border? (F)"=FALSE, "font"=w147, "text"=w142, "start (-1, -1)"=w141, "end (-1, -1)"=w141, "error in (no error)"=w145) -> ("report out"=w140:refnum<class "NI_report.lvclass">, "error out"=w139:errorcluster)  [unwired: 4 in, 3 out]
    n27 = call <vilib>:"Excel Set Cell Alignment.vi"("report in"=w140, "vertical alignment (top)"=w148, "horizontal alignment (left)"=w149, "start (-1, -1)"=w141, "end (-1, -1)"=w141, "error in (no error)"=w139) -> ("report out"=w143:refnum<class "NI_report.lvclass">, "error out"=w146:errorcluster)  [unwired: 8 in]
  }
  n28 = Unbundle By Name("UEF Calculated Values Input") -> ("Sampled Data.Qe (Wh)"=w13:dbl, "Test Information.Rate Input (kW or BTU/hr)"=w55:string, "Test Information.Measured Input (kW or BTU/hr)"=w54:string)
  n29 = call <vilib>:"Excel Easy Text.vi"("report in"=w34, "border? (F)"=FALSE, "font"=w15, "text"=w31, "start (-1, -1)"=w33, "end (-1, -1)"=w33, "error in (no error)"=w35) -> ("report out"=w39:refnum<class "NI_report.lvclass">, "error out"=w40:errorcluster)  [unwired: 4 in, 3 out]
  n30 = call <vilib>:"Excel Set Cell Alignment.vi"("report in"=w39, "vertical alignment (top)"=w38, "horizontal alignment (left)"=w37, "start (-1, -1)"=w33, "end (-1, -1)"=w33, "error in (no error)"=w40) -> ("report out"=w14:refnum<class "NI_report.lvclass">, "error out"=w16:errorcluster)  [unwired: 8 in]
  n31 = Number To Fractional String(number=w13, width (-)=w11, precision (6)=w11) -> (F-format string=w12:string)  [unwired: 1 in]
  n32 = Build Array(w55, w54) -> (w52:string[])
  n33 = call <vilib>:"Excel Easy Text.vi"("report in"=w14, "border? (F)"=FALSE, "font"=w15, "text"=w12, "start (-1, -1)"=w4, "end (-1, -1)"=w4, "error in (no error)"=w16) -> ("report out"=w18:refnum<class "NI_report.lvclass">, "error out"=w17:errorcluster)  [unwired: 4 in, 3 out]
  n34 = call <vilib>:"Excel Set Cell Alignment.vi"("report in"=w18, "vertical alignment (top)"=w19, "horizontal alignment (left)"=w20, "start (-1, -1)"=w4, "end (-1, -1)"=w4, "error in (no error)"=w17) -> ("report out"=w10:refnum<class "NI_report.lvclass">, "error out"=w8:errorcluster)  [unwired: 8 in]
  n35 = call <vilib>:"Excel Set Cell Color and Border.vi"("report in"=w10, "outside border"=w6, "background color (w)"=u32 16777164, "start (-1, -1)"=w4, "end (-1, -1)"=w4, "error in (no error)"=w8) -> ("report out"=w9:refnum<class "NI_report.lvclass">, "error out"=w7:errorcluster)  [unwired: 8 in]
  n36 = case shown="False" w87 {
    tunnel: [u32 16711680 ("background color (w)") u32 45136 ("background color (w)")] -> w88
    frame False {
    }
    frame True {
    }
  }
  n37 = call <vilib>:"Excel Set Cell Color and Border.vi"("report in"=w9, "outside border"=w6, "background color (w)"=w88, "start (-1, -1)"=w86, "end (-1, -1)"=w86, "error in (no error)"=w7) -> ("report out"=w89:refnum<class "NI_report.lvclass">, "error out"=w90:errorcluster)  [unwired: 8 in]
  n38 = call <vilib>:"Excel Set Cell Color and Border.vi"("report in"=w89, "outside border"=w6, "background color (w)"=w88, "start (-1, -1)"=w85, "end (-1, -1)"=w85, "error in (no error)"=w90) -> ("report out"=w83:refnum<class "NI_report.lvclass">, "error out"=w82:errorcluster)  [unwired: 8 in]
  n39 = call <vilib>:"Excel Set Cell Color and Border.vi"("report in"=w83, "outside border"=w6, "start (-1, -1)"=w81, "end (-1, -1)"=w81, "error in (no error)"=w82) -> ("report out"=w65:refnum<class "NI_report.lvclass">, "error out"=w66:errorcluster)  [unwired: 9 in]
  n40 = for {
    tunnel: w59 -> [w163] mode=indexing
    shift-right: [w157] -> w50
    shift-left: w66 -> [w165]
    shift-right: [w158] -> w51
    shift-left: w65 -> [w164]
    tunnel: cluster{"row":i32, "column":i32}[] [{"row"=26, "column"=7}, {"row"=32, "column"=7}, {"row"=33, "column"=7}, {"row"=34, "column"=7}, {"row"=35, "column"=7}, {"row"=32, "column"=12}] -> [w153] mode=indexing
    tunnel: T6 {"font name"="", "font size"=16.0, "bold"=1, "italic"=0, "underline"=0, "strike through"=0, "font color"=16777216} ("font") -> [w160]
    tunnel: w6 -> [w155]
    w167 = 1 items=["left", "center", "right"] ("horizontal alignment (left)")
    w166 = 1 items=["top", "center", "bottom"] ("vertical alignment (top)")
    n41 = call <vilib>:"Excel Easy Text.vi"("report in"=w164, "border? (F)"=FALSE, "font"=w160, "text"=w163, "start (-1, -1)"=w153, "end (-1, -1)"=w153, "error in (no error)"=w165) -> ("report out"=w162:refnum<class "NI_report.lvclass">, "error out"=w161:errorcluster)  [unwired: 4 in, 3 out]
    n42 = call <vilib>:"Excel Set Cell Alignment.vi"("report in"=w162, "vertical alignment (top)"=w166, "horizontal alignment (left)"=w167, "start (-1, -1)"=w153, "end (-1, -1)"=w153, "error in (no error)"=w161) -> ("report out"=w159:refnum<class "NI_report.lvclass">, "error out"=w156:errorcluster)  [unwired: 8 in]
    n43 = call <vilib>:"Excel Set Cell Color and Border.vi"("report in"=w159, "outside border"=w155, "background color (w)"=u32 9810903, "start (-1, -1)"=w153, "end (-1, -1)"=w153, "error in (no error)"=w156) -> ("report out"=w158:refnum<class "NI_report.lvclass">, "error out"=w157:errorcluster)  [unwired: 8 in]
  }
  n44 = for {
    tunnel: cluster{"row":i32, "column":i32}[] [{"row"=16, "column"=16}, {"row"=17, "column"=16}] -> [w169] mode=indexing
    shift-right: [w172] -> w47
    shift-left: w51 -> [w178]
    shift-right: [w171] -> w46
    shift-left: w50 -> [w177]
    tunnel: w52 -> [w175] mode=indexing
    i -> [w170]
    w180 = 0 items=["left", "center", "right"] ("horizontal alignment (left)")
    w181 = 1 items=["top", "center", "bottom"] ("vertical alignment (top)")
    n45 = call <vilib>:"Excel Easy Text.vi"("report in"=w178, "border? (F)"=FALSE, "font"=T6 {"font name"="", "font size"=16.0, "bold"=1, "italic"=0, "underline"=0, "strike through"=0, "font color"=16777216}, "text"=w175, "start (-1, -1)"=w169, "end (-1, -1)"=w169, "error in (no error)"=w177) -> ("report out"=w182:refnum<class "NI_report.lvclass">, "error out"=w183:errorcluster)  [unwired: 4 in, 3 out]
    n46 = call <vilib>:"Excel Set Cell Alignment.vi"("report in"=w182, "vertical alignment (top)"=w181, "horizontal alignment (left)"=w180, "start (-1, -1)"=w169, "end (-1, -1)"=w169, "error in (no error)"=w183) -> ("report out"=w173:refnum<class "NI_report.lvclass">, "error out"=w174:errorcluster)  [unwired: 8 in]
    n47 = case shown="1" w170 {
      tunnel: w174 -> [w184 w190]
      tunnel: w173 -> [w185 w189]
      tunnel: [w185 w188] -> w172
      tunnel: [w184 w187] -> w171
      tunnel: w169 -> [_ w186]
      frame 0, Default {
      }
      frame 1 {
        n48 = call <vilib>:"Excel Set Cell Color and Border.vi"("report in"=w189, "background color (w)"=u32 9286882, "start (-1, -1)"=w186, "end (-1, -1)"=w186, "error in (no error)"=w190) -> ("report out"=w188:refnum<class "NI_report.lvclass">, "error out"=w187:errorcluster)  [unwired: 9 in]
      }
    }
  }
  n49 = Build Array(w43, w42) -> (w41:string[])
  n50 = for {
    tunnel: cluster{"row":i32, "column":i32}[] [{"row"=74, "column"=8}, {"row"=75, "column"=8}] -> [w192] mode=indexing
    shift-right: [w195] -> w45
    shift-left: w47 -> [w201]
    shift-right: [w194] -> w44
    shift-left: w46 -> [w200]
    tunnel: w41 -> [w198] mode=indexing
    i -> [w193]
    w203 = 0 items=["left", "center", "right"] ("horizontal alignment (left)")
    w204 = 1 items=["top", "center", "bottom"] ("vertical alignment (top)")
    n51 = call <vilib>:"Excel Easy Text.vi"("report in"=w201, "border? (F)"=FALSE, "font"=T6 {"font name"="", "font size"=16.0, "bold"=1, "italic"=0, "underline"=0, "strike through"=0, "font color"=16777216}, "text"=w198, "start (-1, -1)"=w192, "end (-1, -1)"=w192, "error in (no error)"=w200) -> ("report out"=w205:refnum<class "NI_report.lvclass">, "error out"=w206:errorcluster)  [unwired: 4 in, 3 out]
    n52 = call <vilib>:"Excel Set Cell Alignment.vi"("report in"=w205, "vertical alignment (top)"=w204, "horizontal alignment (left)"=w203, "start (-1, -1)"=w192, "end (-1, -1)"=w192, "error in (no error)"=w206) -> ("report out"=w196:refnum<class "NI_report.lvclass">, "error out"=w197:errorcluster)  [unwired: 8 in]
    n53 = case shown="1" w193 {
      tunnel: w197 -> [w207 w214]
      tunnel: w196 -> [w208 w213]
      tunnel: [w208 w212] -> w195
      tunnel: [w207 w211] -> w194
      tunnel: w192 -> [_ w210]
      frame 0, Default {
      }
      frame 1 {
        n54 = call <vilib>:"Excel Set Cell Color and Border.vi"("report in"=w213, "background color (w)"=u32 16777215, "start (-1, -1)"=w210, "end (-1, -1)"=w210, "error in (no error)"=w214) -> ("report out"=w212:refnum<class "NI_report.lvclass">, "error out"=w211:errorcluster)  [unwired: 9 in]
      }
    }
  }
  "error out" <- w44
  "report out" <- w45
